vi "MatrixTest.vi"() -> ()   [LabVIEW 2020]
panel:
  in  "pattern in":u32[](array[numeric])
  out "pattern out":u32[](array[numeric])
  out "error out":errorcluster={"status"=FALSE, "code"=0, "source"="pipx40 Close.vi"}
  in  "RUN/ STOP":bool
  in  "Open":bool
  in  "Row":i32=1 min=1
  in  "Column":i32=1 min=1
  in  "VISA resource name":refnum<visa-resource-name>="PXI14::13::INSTR"
  out "Model Name":string="Pickering 40-523-022"
  out "ID String":string="PICKERING INTERFACES,40-523-022,210512,1.01"
  out "Number of Columns":i32=44
  out "Number of Rows":i32=4
  in  "Sub Unit Number":i32=1 min=1
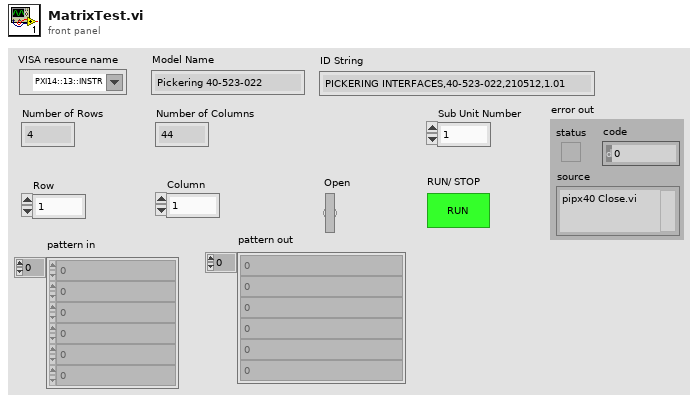
[diagram p1: front panel]
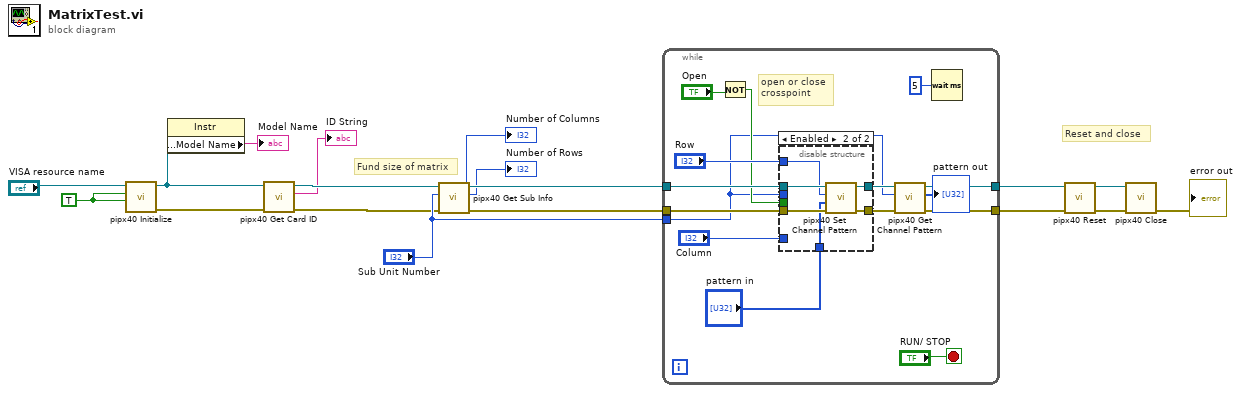
[diagram p0: block diagram]
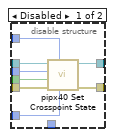
[diagram p2: hidden frame]
diagram:
  w12 = TRUE
  # "Reset and close"
  # "Fund size of matrix"
  n1 = call <instrlib>:"pipx40 Initialize.vi"("reset device"=w12, "id query"=w12, "resource name"="VISA resource name") -> ("error out"=w11:errorcluster, "instrument handle out"=w6:refnum<visa-resource-name>)  [unwired: 7 in]
  n2 = property on="Property Node" class="Instr"(reference=w6) -> ("General Settings:Model Name"=→"Model Name":string)  [unwired: 1 in, 2 out]
  n3 = call <instrlib>:"pipx40 Get Card ID.vi"("error in (no error)"=w11, "instrument handle"=w6) -> ("error out"=w8:errorcluster, "id string"=→"ID String":string, "instrument handle out"=w9:refnum<visa-resource-name>)  [unwired: 7 in]
  n4 = call <instrlib>:"pipx40 Get Sub Info.vi"("error in (no error)"=w8, "subunit number"="Sub Unit Number", "instrument handle"=w9) -> ("error out"=w17:errorcluster, "columns"=→"Number of Columns":u32, "rows"=→"Number of Rows":u32, "instrument handle out"=w18:refnum<visa-resource-name>)  [unwired: 4 in, 1 out]
  n5 = while {
    tunnel: "Sub Unit Number" -> [w21]
    tunnel: w17 -> [w30]
    tunnel: w18 -> [w29]
    tunnel: [w22] -> w15
    tunnel: [w23] -> w14
    stop <- "RUN/ STOP" stop-if-true
    # "open or close\ncrosspoint"
    n6 = Not(x="Open") -> (.not. x?=w27:bool)
    n7 = disable-structure shown="Enabled" {
      disable-tunnel: "Row" -> [w41 w43]
      disable-tunnel: "Column" -> [w40 _]
      disable-tunnel: w30 -> [w39 w47]
      disable-tunnel: w29 -> [w38 w44]
      disable-tunnel: w27 -> [w37 _]
      disable-tunnel: [w36 w46] -> w25
      disable-tunnel: [w35 w45] -> w24
      disable-tunnel: w21 -> [w34 _]
      disable-tunnel: "pattern in" -> [_ w42]
      frame Disabled {
        n8 = call <instrlib>:"pipx40 Set Crosspoint State.vi"("column location"=w40, "row location"=w41, "error in (no error)"=w39, "action"=w37, "subunit number"=w34, "instrument handle"=w38) -> ("error out"=w36:errorcluster, "instrument handle out"=w35:refnum<visa-resource-name>)  [unwired: 4 in]
      }
      frame Enabled {
        n9 = call <instrlib>:"pipx40 Set Channel Pattern.vi"("error in (no error)"=w47, "pattern"=w42, "subunit number"=w43, "instrument handle"=w44) -> ("error out"=w46:errorcluster, "instrument handle out"=w45:refnum<visa-resource-name>)  [unwired: 6 in]
      }
    }
    n10 = call <instrlib>:"pipx40 Get Channel Pattern.vi"("error in (no error)"=w25, "subunit number"=w21, "instrument handle"=w24) -> ("error out"=w23:errorcluster, "pattern"=→"pattern out":u32[], "instrument handle out"=w22:refnum<visa-resource-name>)  [unwired: 6 in]
    n11 = Wait (ms)(milliseconds to wait=u32 5) -> ()  [unwired: 1 out]
  }
  n12 = call <instrlib>:"pipx40 Reset.vi"("error in (no error)"=w14, "instrument handle"=w15) -> ("error out"=w2:errorcluster, "instrument handle out"=w3:refnum<visa-resource-name>)  [unwired: 8 in]
  n13 = call <instrlib>:"pipx40 Close.vi"("error in (no error)"=w2, "instrument handle"=w3) -> ("error out"=→"error out":errorcluster)  [unwired: 9 in]
